vi "executeKeeperPlay.vi"(8 "error in (no error)":errorcluster, 11 "Game in":refnum<class "Game.lvclass">) -> (0 "error out":errorcluster, 3 "Game out":refnum<class "Game.lvclass">)   [LabVIEW 2018, in "Game.lvclass"]
uses:
  Game.lvclass
  Game.lvclass/Game.ctl
  Team_class/Team.lvclass/Team.ctl
  Playbook_class/Playbook.lvclass/Playbook.ctl
  TestPlay_class/TestPlay.lvclass/TestPlay.ctl
  Playbook_class/Read keeper_plays.vi
  TestPlay_class/Read Roles.vi
  Read KeeperTeam.vi
  Read Playbook.vi
  Team_class/Read RobotRef.vi
  Team_class/Read KeeperPlay.vi
  Team_class/Write RobotRef.vi
  Write KeeperTeam.vi
  Ally_class/Ally.lvclass
  C:/Users/Rebeca/Documents/Rebeca/Roboime/SSL_AI/Team_class/Team.lvclass
  Playbook_class/Playbook.lvclass
  Robot_class/Robot.lvclass
  Play_class/Play.lvclass
  TestPlay_class/TestPlay.lvclass
  HaltPlay_class/HaltPlay.lvclass
  KeeperPlay_class/KeeperPlay.lvclass
  TestRole_class/TestRole.lvclass
  Role_class/Role.lvclass
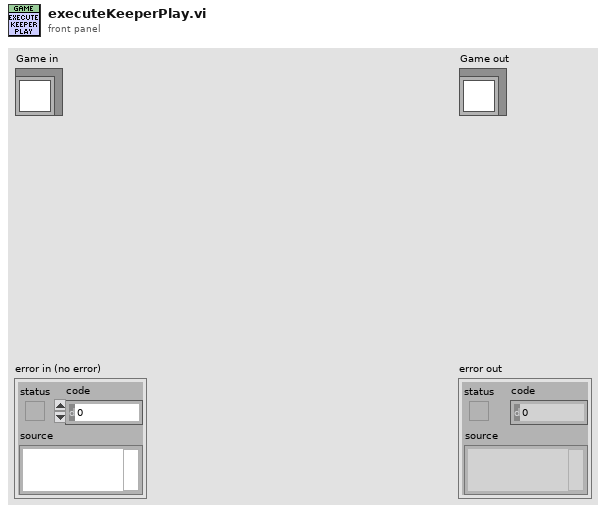
[diagram p1: front panel]
types:
  T1 = typedef "KeeperPlay.ctl" = enum16{"NormalGame", "KeeperPlay", "Halt", "Timeout", "PenaltyEnemy", "TestPlay"}
  T2 = cluster{"Play":refnum<class "Play.lvclass">, "TestPlay":refnum<class "TestPlay.lvclass">, "HaltPlay":refnum<class "HaltPlay.lvclass">, "KeeperPlay":refnum<class "KeeperPlay.lvclass">}
  T3 = cluster{"TestRole 1":refnum<class "TestRole.lvclass">, "Role":refnum<class "Role.lvclass">, "TestRole 2":refnum<class "TestRole.lvclass">, "TestRole 3":refnum<class "TestRole.lvclass">}
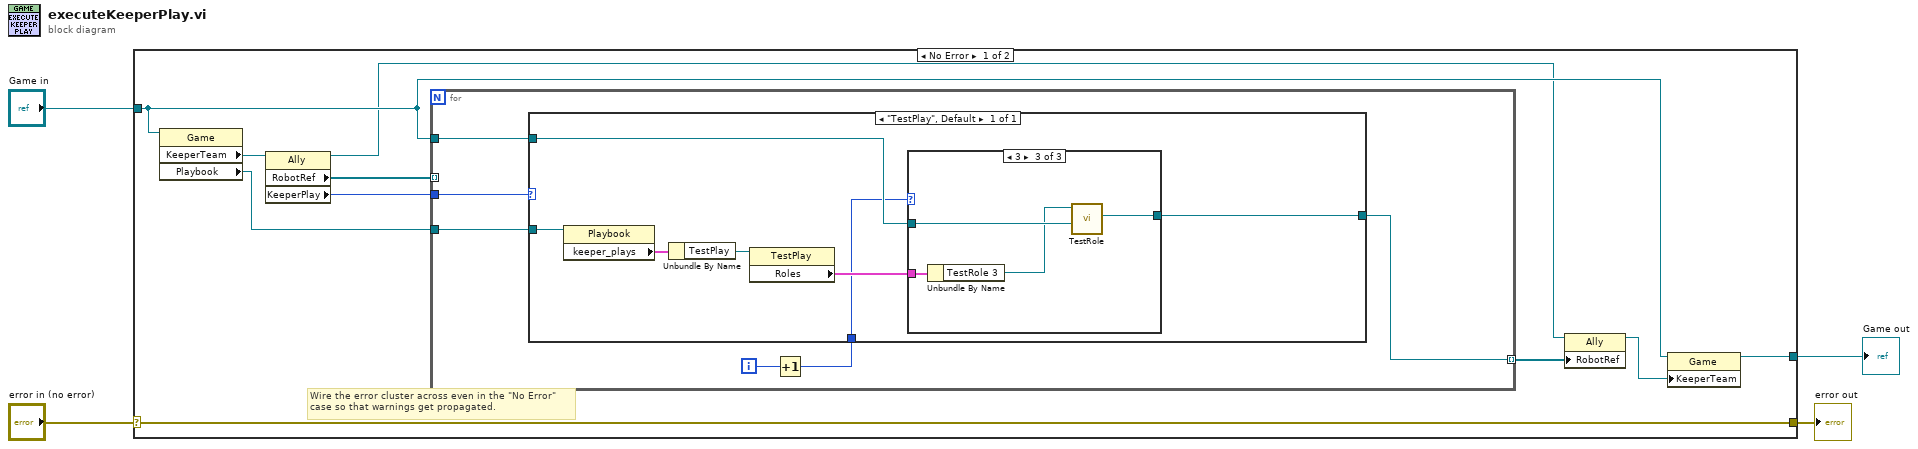
[diagram p0: block diagram]
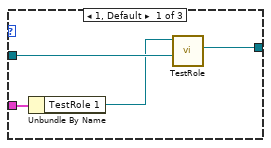
[diagram p2: hidden frame]
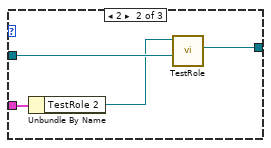
[diagram p3: hidden frame]
diagram:
  n1 = case shown="No Error" "error in (no error)" {
    selector: "error in (no error)" -> [w14 w41]
    tunnel: [w14 w41] -> w3
    tunnel: [w6 w40] -> w1
    tunnel: "Game in" -> [w9 w40]
    frame No Error {
      # "Wire the error cluster across even in the \"No Error\"\ncase so that warnings get propagated."
      n2 = property class="Game"(reference=w9) -> ("KeeperTeam"=w13:refnum<class "Ally.lvclass">, "Playbook"=w10:refnum<class "Playbook.lvclass">)  [unwired: 1 in, 2 out]
      n3 = property class="Ally"(reference=w13) -> (reference out=w8:refnum<class "Ally.lvclass">, "RobotRef"=w12:refnum<class "Robot.lvclass">[], "KeeperPlay"=w11:T1)  [unwired: 1 in, 1 out]
      n4 = for {
        tunnel: w12 -> [_] mode=indexing
        tunnel: w11 -> [w20]
        tunnel: w10 -> [w19]
        tunnel: w9 -> [w18]
        tunnel: [w17] -> w7 mode=indexing
        i -> [w16]
        n5 = Increment(x=w16) -> (x+1=w15:i32)
        n6 = case shown="\"TestPlay\", Default" w20 {
          tunnel: w19 -> [w27]
          tunnel: w18 -> [w23]
          tunnel: [w22] -> w17
          tunnel: w15 -> [w21]
          frame "TestPlay", Default {
            n7 = property class="Playbook"(reference=w27) -> ("keeper_plays"=w26:T2)  [unwired: 1 in, 2 out]
            n8 = Unbundle By Name(w26) -> ("TestPlay"=w25:refnum<class "TestPlay.lvclass">)
            n9 = property class="TestPlay"(reference=w25) -> ("Roles"=w24:T3)  [unwired: 1 in, 2 out]
            n10 = case shown="3" w21 {
              tunnel: w24 -> [w31 w35 w39]
              tunnel: w23 -> [w30 w34 w38]
              tunnel: [w29 w33 w37] -> w22
              frame 1, Default {
                n11 = Unbundle By Name(w31) -> ("TestRole 1"=w28:refnum<class "TestRole.lvclass">)
                n12 = call-dynamic "TestRole.vi"("Game in"=w30, "TestRole in"=w28) -> ("Robot out"=w29:refnum<class "Robot.lvclass">)  [unwired: 6 in, 3 out]
              }
              frame 2 {
                n13 = Unbundle By Name(w35) -> ("TestRole 2"=w32:refnum<class "TestRole.lvclass">)
                n14 = call-dynamic "TestRole.vi"("Game in"=w34, "TestRole in"=w32) -> ("Robot out"=w33:refnum<class "Robot.lvclass">)  [unwired: 6 in, 3 out]
              }
              frame 3 {
                n15 = Unbundle By Name(w39) -> ("TestRole 3"=w36:refnum<class "TestRole.lvclass">)
                n16 = call-dynamic "TestRole.vi"("Game in"=w38, "TestRole in"=w36) -> ("Robot out"=w37:refnum<class "Robot.lvclass">)  [unwired: 6 in, 3 out]
              }
            }
          }
        }
      }
      n17 = property class="Ally"(reference=w8, "RobotRef"=w7) -> (reference out=w5:refnum<class "Ally.lvclass">)  [unwired: 1 in, 1 out]
      n18 = property class="Game"(reference=w9, "KeeperTeam"=w5) -> (reference out=w6:refnum<class "Game.lvclass">)  [unwired: 1 in, 1 out]
    }
    frame Error {
    }
  }
  "error out" <- w3
  "Game out" <- w1
